vi "ThreeWaySwitchTest.vi"() -> ()   [LabVIEW 2012]
panel:
  out "Sync2 2":bool
  out "Sync1 2":bool
  out "Sync0 2":bool
  in  "stop":bool
  in  "Sync0":bool
  in  "Sync1":bool
  in  "Sync2":bool
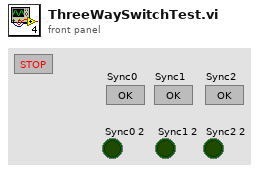
[diagram p1: front panel]
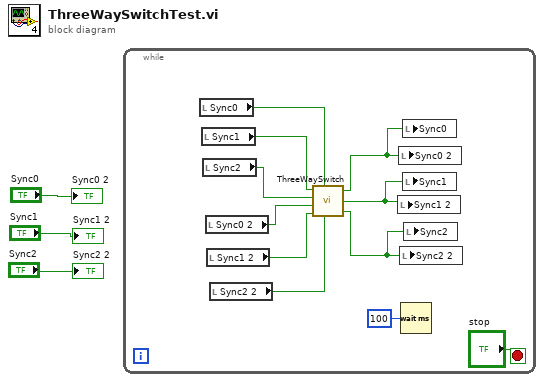
[diagram p0: block diagram]
diagram:
  n1 = while {
    stop <- "stop" stop-if-true
    n2 = local read "Sync0"() -> (w7:bool)
    n3 = local read "Sync1"() -> (w6:bool)
    n4 = local read "Sync2"() -> (w5:bool)
    n5 = local read "Sync0 2"() -> (w13:bool)
    n6 = local read "Sync1 2"() -> (w12:bool)
    n7 = local read "Sync2 2"() -> (w11:bool)
    n8 = call "ThreeWaySwitch.vi"("Sync1"=w6, "Sync0"=w7, "Sync2"=w5, "Sync0 last state"=w13, "Sync2 last state"=w11, "Sync1 last state"=w12) -> ("Sync0out"=w9:bool, "Sync1out"=w10:bool, "Sync2out"=w8:bool)
    n9 = local write "Sync1 2"(w10) -> ()
    n10 = local write "Sync0 2"(w9) -> ()
    n11 = local write "Sync2 2"(w8) -> ()
    n12 = Wait (ms)(milliseconds to wait=u32 100) -> ()  [unwired: 1 out]
    n13 = local write "Sync0"(w9) -> ()
    n14 = local write "Sync1"(w10) -> ()
    n15 = local write "Sync2"(w8) -> ()
  }
  "Sync0 2" <- "Sync0"
  "Sync1 2" <- "Sync1"
  "Sync2 2" <- "Sync2"
